vi "Something_working.vi"() -> ()   [LabVIEW 2014]
doc: "Use this template to simulate the generation and display of data.\nNote: LabVIEW enables automatic error handling by default for VIs you create from this template."
panel:
  in  "On/Off":bool=TRUE caption="stop (T)"
  out "data":dynamicdata(graph)
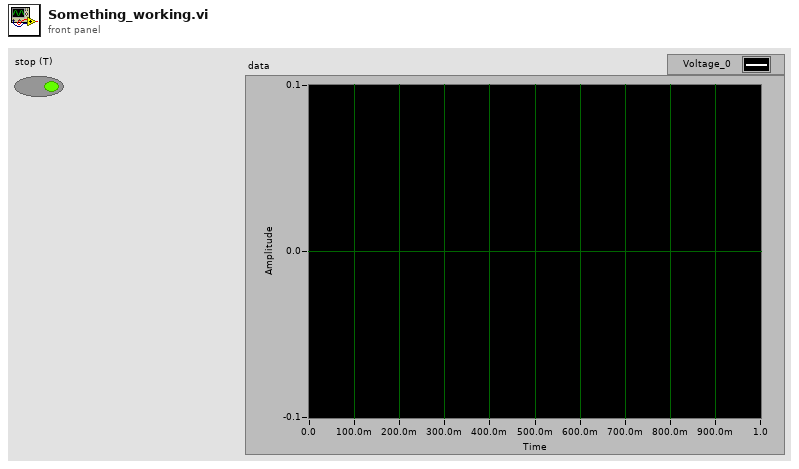
[diagram p1: front panel]
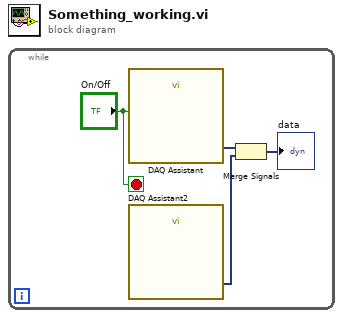
[diagram p0: block diagram]
diagram:
  n1 = while {
    stop <- "On/Off" stop-if-true
    n2 = call "DAQ Assistant"("stop (T)"="On/Off") -> ("data"=w4:dynamicdata)  [unwired: 16 in, 2 out]
    n3 = call "DAQ Assistant2"() -> ("data"=w1:dynamicdata)  [unwired: 17 in, 2 out]
    n4 = Merge Signals(w4, w1) -> (→"data":dynamicdata)
  }
